vi "2 Button Dialog Box.vi"(6 "error in":errorcluster, 7 "button 2 text":string, 8 "button 1 text":string, 9 "Message":string="LOGIN STATUS......") -> (0 "error out":errorcluster, 2 "button pressed?":string, 3 "Message":string)   [LabVIEW 2015]
panel:
  in  "stop":bool
  in  "Title":string="Confirmation STATUS......"
  in  "button 2":bool
  in  "button 1":bool
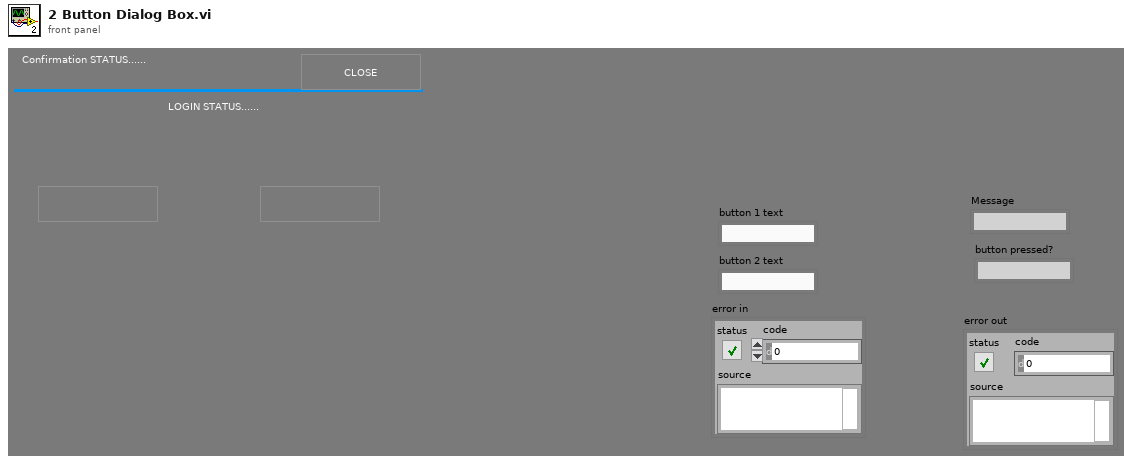
[diagram p1: front panel]
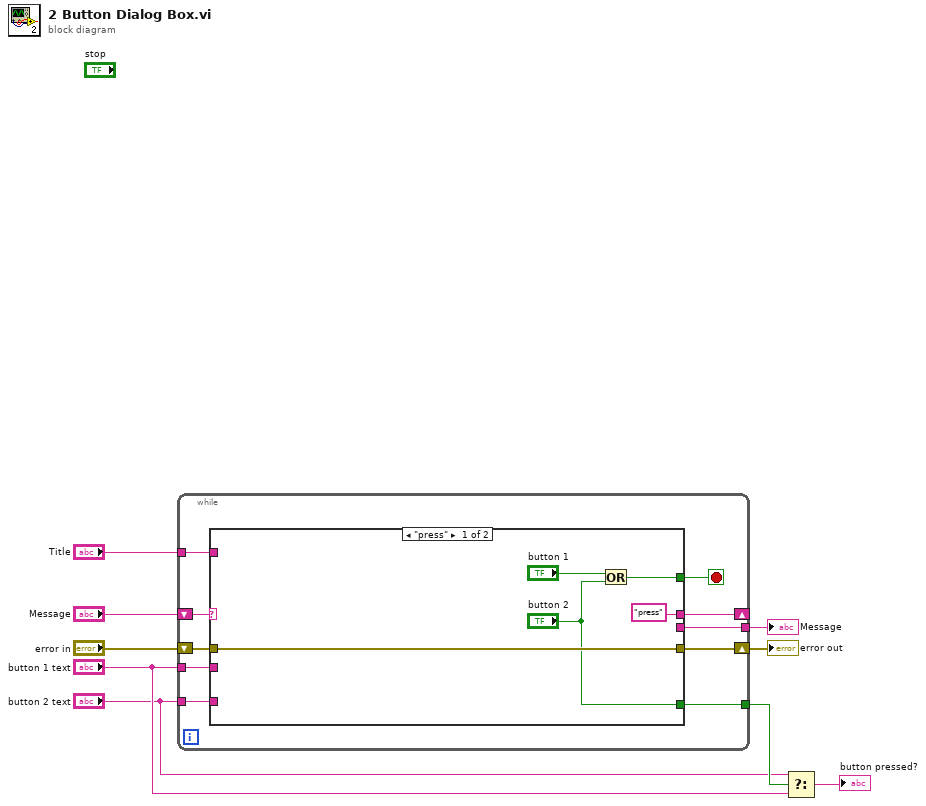
[diagram p0: block diagram]
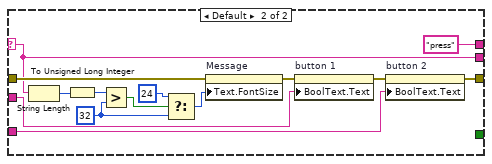
[diagram p2: hidden frame]
diagram:
  n1 = while {
    shift-right: [w19] -> _
    shift-left: "Message" -> [w18]
    tunnel: "button 1 text" -> [w17]
    tunnel: [w14] -> w7
    tunnel: "button 2 text" -> [w12]
    tunnel: [w11] -> w5
    tunnel: "Title" -> [w10]
    shift-right: [w15] -> w6
    shift-left: "error in" -> [w16]
    stop <- w13 stop-if-true
    n2 = case shown="\"press\"" w18 {
      selector: w18 -> [_ w25]
      tunnel: w10 -> [_ _]
      tunnel: w17 -> [_ w37]
      tunnel: [w22 _] -> w13
      tunnel: ["press" "press"] -> w19
      tunnel: w16 -> [w23 w28]
      tunnel: [w23 w35] -> w15
      tunnel: [_ w25] -> w14
      tunnel: w12 -> [_ w34]
      tunnel: ["button 2" _] -> w11
      frame "press" {
        n3 = Or(x="button 1", y="button 2") -> (x .or. y?=w22:bool)
      }
      frame Default {
        w26 = u32 32 ("y")
        n4 = String Length(string=w25) -> (length=w31:i32)
        n5 = To Unsigned Long Integer(number=w31) -> (unsigned 32bit integer=w30:u32)
        n6 = Greater?(x=w30, y=w26) -> (0:w33:bool)
        n7 = Select(t=u32 24, s=w33, f=w26) -> (s? t:f=w29:u32)
        n8 = property on="Message" class="Str"(error in=w28, "Text.FontSize"=w29) -> (error out=w27:errorcluster)  [unwired: 1 in, 1 out]
        n9 = property on="button 1" class="Bool"(error in=w27, "BoolText.Text"=w37) -> (error out=w36:errorcluster)  [unwired: 1 in, 1 out]
        n10 = property on="button 2" class="Bool"(error in=w36, "BoolText.Text"=w34) -> (error out=w35:errorcluster)  [unwired: 1 in, 1 out]
      }
    }
  }
  "Message" <- w7
  "error out" <- w6
  n11 = Select(t="button 2 text", s=w5, f="button 1 text") -> (s? t:f=→"button pressed?":string)
